vi "relative access path.vi"(11 "Oauth2.Slack":refnum<class "Oauth2.Slack.lvclass">) -> (1 "Token Access Path":string, 2 "Authorization Path":string)   [LabVIEW 2020, in "Oauth2.Slack.lvclass"]
uses:
  Oauth2.Slack.lvclass
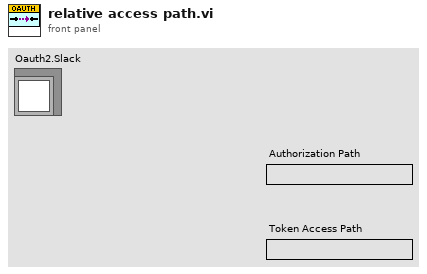
[diagram p1: front panel]
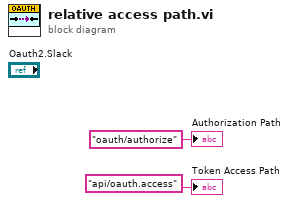
[diagram p0: block diagram]
diagram:
  "Authorization Path" <- "oauth/authorize" ("Authorization Path")
  "Token Access Path" <- "api/oauth.access" ("Authorization Path")
